vi "Tabulate_FFID_Bkgnd_Volts.vi"() -> ()   [LabVIEW 2011]
uses:
  Controls/Post_Process.ctl
  Controls/Setup.ctl
  Controls/Save_Data.ctl
  Globals/Meas_global.vi
  Controls/File_Selector_Type.ctl
panel:
  in  "At Dialog Prompt Post Process":T1=enum."Files containing the search string in the selected folder"
  in  "Search String":string="FF_Bkgnd_"
  out "current index":i32
  out "No Of files":i32
  in  "Raw Data folder":path
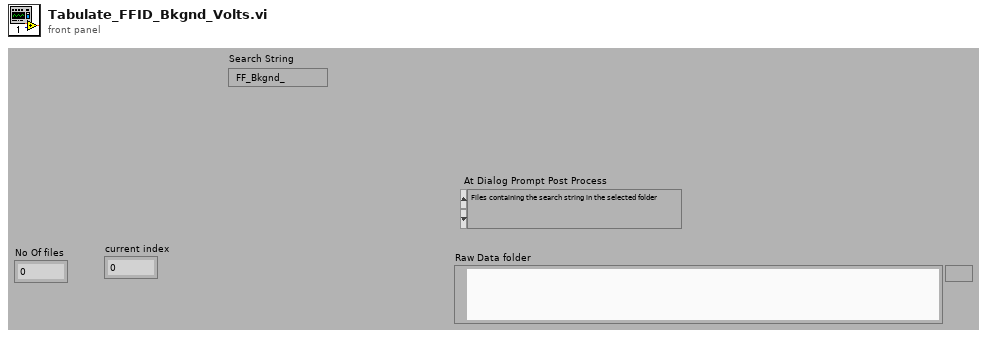
[diagram p1: front panel]
types:
  T1 = typedef "File_Selector_Type.ctl" = enum16{"The Selected File", "The Selected Folder", "Files containing the search string in the selected folder", "All files listed in selected file"}
  T2 = typedef "Save_Data.ctl" = enum16{"Save No Data", "Save Data"}
  T3 = typedef "Setup.ctl" = enum16{"Run Program", "Show Setup", "Save Current Setup", "Setup Front Panel"}
  T4 = typedef "Post_Process.ctl" = enum16{"Take New Data", "Post Process Raw Data File"}
  T5 = typedef "Analysis_info_cluster.ctl" = cluster{"Colour":u32, "Inst type":T6, "Inst name":string, "Symbol":string, "Code name":string, "Extra Info":string, "Inst Array":T7, "Index":i32, "Voltage Index":i32, "Extra Titles":string[], "Extra Values":string[], "Eng Values":dbl[], "Time (ms)":dbl[], "Voltage":dbl[], "U":dbl, "u^2":dbl, "u^3":dbl, "u^4":dbl, "Skew_u":dbl, "Kurt_u":dbl, "Sd Error in Mean":dbl, "% u'/U":dbl, "X":dbl, "Y":dbl, "Z":dbl, "Spectra":T8, "Autocorrelation":T8, "Timescale integral to 25%":dbl, "Sd Error in Variance":dbl, "Calib File":path, "Calib Constants":dbl[], "Histogram":T8, "Output Position":bool, "Full Stats":bool, "Weighting":dbl[]}
  T6 = typedef "Inst_type.ctl" = enum16{"Propeller anemometer", "Raw voltage", "Pressure Transducer", "Pitot-static tube", "Preston tube", "Hot wire", "Cross wire 1", "Cross wire 2", "Generic Linear", "Generic Polynomial", "Generic BackPoly", "Fast FID", "Thermocouple", "Cold wire", "Pulsed Wire", "LDA Vel", "LDA Tran time", "LDA Arr time"}
  T7 = typedef "Instrument_Array.ctl" = enum16{"PWA", "LDA", "Analogue"}
  T8 = typedef "XY_Plot_Cluster.ctl" = cluster{"First Name":string, "Second Name":string, "X axis name":string, "Y axis name":string, "X array":dbl[], "Y array":dbl[]}
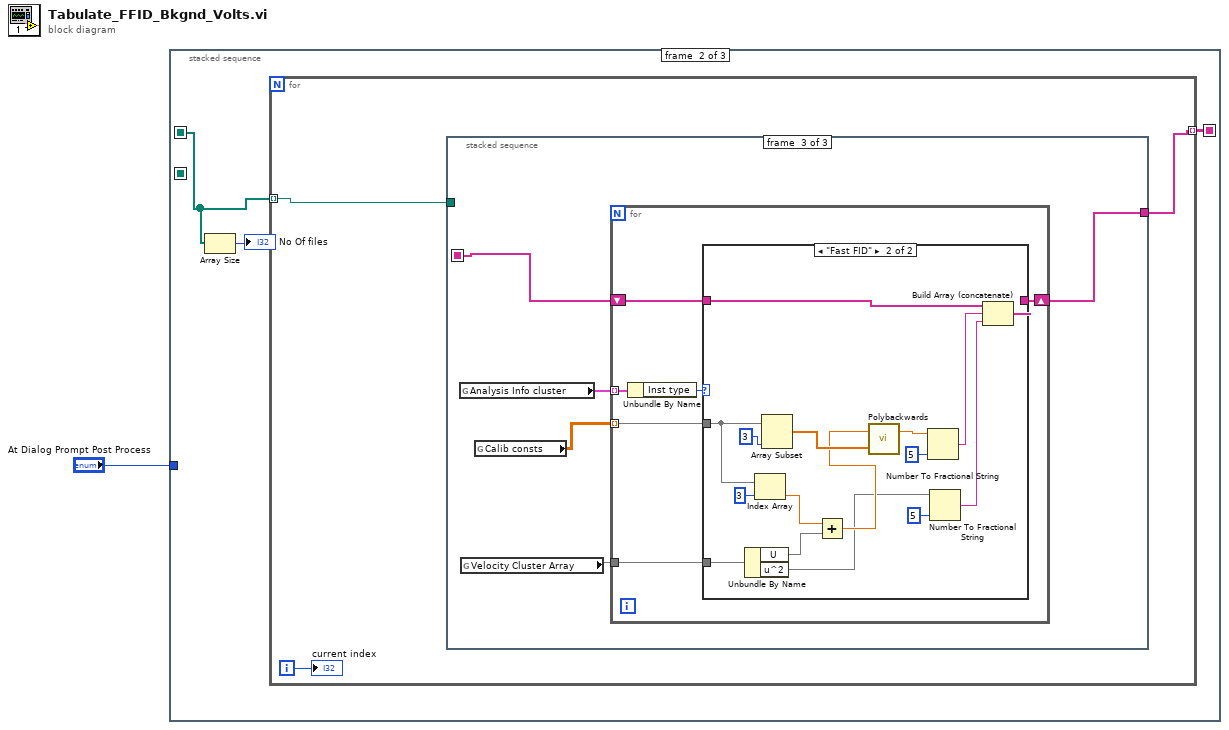
[diagram p0: block diagram]
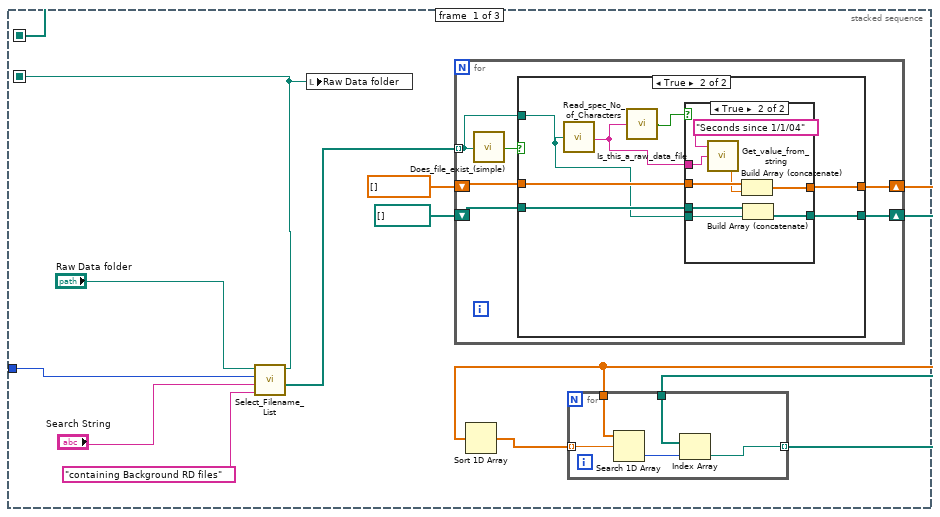
[diagram p2: hidden frame]
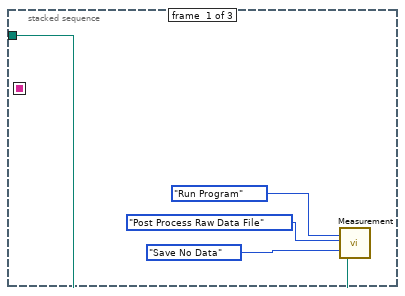
[diagram p5: hidden frame]
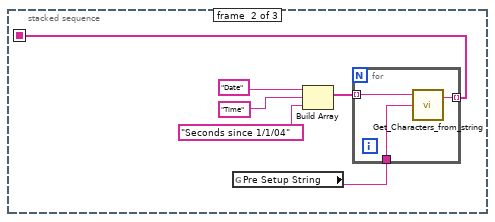
[diagram p6: hidden frame]
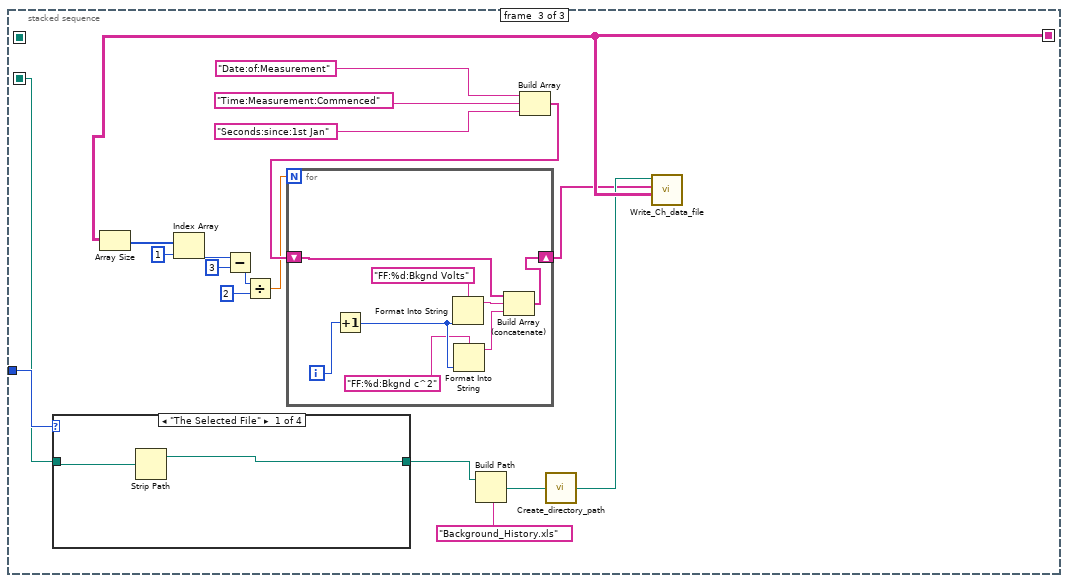
[diagram p8: hidden frame]
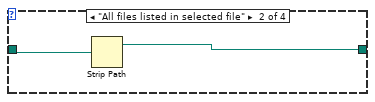
[diagram p9: hidden frame]
diagram:
  n1 = stacked-sequence {
    seq-local: [_ w44 _] -> [_ _ w102]
    seq-local: [w10 _ _] -> [_ _ w96]
    seq-local: [w3 _ _] -> [_ w45 _]
    tunnel: "At Dialog Prompt Post Process" -> [w2 _ w98]
    frame #0 {
      n2 = call "Select_Filename_List.vi"("File Type"="containing Background RD files", "Search String"="Search String", "At Dialog Prompt Post Process"=w2, "Previous Choice"="Raw Data folder") -> ("Selected files"=w4:path[], "Choosen path"=w10:path)  [unwired: 1 in, 2 out]
      n3 = local write "Raw Data folder"(w10) -> ()
      n4 = for {
        tunnel: w4 -> [w19] mode=indexing
        shift-right: [w23] -> w5
        shift-left: dbl[] [] -> [w24]
        shift-right: [w21] -> w8
        shift-left: path[] [] -> [w22]
        n5 = call "Does_file_exist_(simple).vi"("Pathname"=w19) -> ("exists?"=w20:bool)
        n6 = case shown="True" w20 {
          tunnel: w24 -> [w26 w33]
          tunnel: [w26 w32] -> w23
          tunnel: w22 -> [w25 w31]
          tunnel: [w25 w30] -> w21
          tunnel: w19 -> [_ w28]
          frame False {
          }
          frame True {
            n7 = call "Read_spec_No_of_Characters.vi"("Filename"=w28) -> ("character string"=w27:string)  [unwired: 1 out]
            n8 = call "Is_this_a_raw_data_file.vi"("character string"=w27) -> ("Raw Dat File?"=w29:bool)  [unwired: 2 out]
            n9 = case shown="True" w29 {
              tunnel: w33 -> [w35 w41]
              tunnel: [w35 w43] -> w32
              tunnel: w31 -> [w34 w39]
              tunnel: w28 -> [_ w38]
              tunnel: [w34 w37] -> w30
              tunnel: w27 -> [_ w36]
              frame False {
              }
              frame True {
                n10 = call "Get_value_from_string.vi"("Input string"=w36, "Variable name"="Seconds since 1/1/04") -> ("Value"=w40:dbl)  [unwired: 1 in, 1 out]
                n11 = Build Array (concatenate)(w41, w40) -> (w43:dbl[])
                n12 = Build Array (concatenate)(w39, w38) -> (w37:path[])
              }
            }
          }
        }
      }
      n13 = Sort 1D Array(array=w5) -> (sorted array=w6:dbl[])
      n14 = for {
        tunnel: w5 -> [w18]
        tunnel: w6 -> [w17] mode=indexing
        tunnel: w8 -> [w16]
        tunnel: [w15] -> w3 mode=indexing
        n15 = Search 1D Array(1D array=w18, element=w17) -> (index of element=w14:i32)  [unwired: 1 out]
        n16 = Index Array(array=w16, index=w14) -> (element=w15:path)
      }
    }
    frame #1 {
      n17 = Array Size(array=w45) -> (size(s)=→"No Of files":i32)
      n18 = for {
        tunnel: w45 -> [w49] mode=indexing
        tunnel: [w47] -> w44 mode=indexing
        i -> [w48]
        n19 = stacked-sequence {
          seq-local: [_ w54 _] -> [_ _ w64]
          tunnel: w49 -> [w50 _ _]
          tunnel: [_ _ w63] -> w47
          frame #0 {
            n20 = call "Measurement.vi"("setup"=Setup."Run Program", "Post Process"=Post_Process."Post Process Raw Data File", "File"=Save_Data."Save No Data", "Raw data file"=w50) -> ()  [unwired: 3 in, 13 out]
          }
          frame #1 {
            n21 = global read "Meas_global.vi" "Pre Setup String"() -> (w55:string)
            n22 = Build Array("Date", "Time", "Seconds since 1/1/04") -> (w56:string[])
            n23 = for {
              tunnel: w56 -> [w62] mode=indexing
              tunnel: w55 -> [w61]
              tunnel: [w60] -> w54 mode=indexing
              n24 = call "Get_Characters_from_string.vi"("Input string"=w61, "Variable name"=w62) -> ("Value"=w60:string)  [unwired: 1 in, 1 out]
            }
          }
          frame #2 {
            n25 = global read "Meas_global.vi" "Analysis Info cluster"() -> (w67:T5[])
            n26 = global read "Meas_global.vi" "Velocity Cluster Array"() -> (w65)
            n27 = global read "Meas_global.vi" "Calib consts"() -> (w66:dbl[][])
            n28 = for {
              tunnel: w67 -> [w73] mode=indexing
              tunnel: w66 -> [w72] mode=indexing
              tunnel: w65 -> [w70]
              shift-right: [w68] -> w63
              shift-left: w64 -> [w69]
              n29 = Unbundle By Name(w73) -> ("Inst type"=w71:T6)
              n30 = case shown="\"Fast FID\"" w71 {
                tunnel: w72 -> [_ w85]
                tunnel: w70 -> [_ w84]
                tunnel: w69 -> [w74 w81]
                tunnel: [w74 w78] -> w68
                frame "Propeller anemometer", Default {
                }
                frame "Fast FID" {
                  n31 = Unbundle By Name(w84) -> ("U"=w87, "u^2"=w75)
                  n32 = Index Array(array=w85, index=3 ("Index")) -> (element=w86:dbl)
                  n33 = Array Subset(array=w85, length=3 ("index")) -> (w90:dbl[])  [unwired: 1 in]
                  n34 = Add(x=w86, y=w87) -> (x+y=w83:dbl)
                  n35 = call "Polybackwards.vi"("Coefficients"=w90, "Y input"=w83) -> ("X output"=w79:dbl)  [unwired: 1 out]
                  n36 = Number To Fractional String(number=w79, precision (6)=i16 5) -> (F-format string=w80:string)  [unwired: 2 out]
                  n37 = Number To Fractional String(number=w75, precision (6)=i16 5) -> (F-format string=w76:string)  [unwired: 2 out]
                  n38 = Build Array (concatenate)(w81, w80, w76) -> (w78:string[])
                }
              }
            }
          }
        }
        "current index" <- w48
      }
    }
    frame #2 {
      n39 = case shown="\"The Selected File\"" w98 {
        tunnel: [w110 w112 w114 w115] -> w97
        tunnel: w96 -> [w111 w113 w114 w115]
        frame "The Selected File" {
          n40 = Strip Path(path=w111) -> (stripped path=w110:path)  [unwired: 1 out]
        }
        frame "All files listed in selected file" {
          n41 = Strip Path(path=w113) -> (stripped path=w112:path)  [unwired: 1 out]
        }
        frame "Files containing the search string in the selected folder" {
        }
        frame "The Selected Folder" {
        }
      }
      n42 = Array Size(array=w102) -> (size(s)=w109:i32[])
      n43 = Index Array(array=w109, index=1) -> (element=w103:i32)
      n44 = Subtract(x=w103, y=3) -> (x-y=w93:i32)
      n45 = Divide(x=w93, y=2) -> (x/y=w92:dbl)
      n46 = Build Path(base path=w97, name or relative path="Background_History.xls") -> (appended path=w100:path)
      n47 = Build Array("Date:of:Measurement", "Time:Measurement:Commenced", "Seconds:since:1st Jan") -> (w95:string[])
      n48 = for {
        N: w92 -> [_]
        shift-right: [w117] -> w94
        shift-left: w95 -> [w118]
        i -> [w123]
        n49 = Increment(x=w123) -> (x+1=w121:i32)
        n50 = Format Into String(format string="FF:%d:Bkgnd Volts", w121) -> (resulting string=w120:string)  [unwired: 2 in, 1 out]
        n51 = Format Into String(format string="FF:%d:Bkgnd c^2", w121) -> (resulting string=w119:string)  [unwired: 2 in, 1 out]
        n52 = Build Array (concatenate)(w118, w120, w119) -> (w117:string[])
      }
      n53 = call "Create_directory_path.vi"("Path name"=w100) -> ("Path name Out"=w99:path)
      n54 = call "Write_Ch_data_file.vi"("Channel Values"=w102, "Channel names"=w94, "Filename"=w99) -> ()  [unwired: 5 in, 4 out]
    }
  }
